vi "Check Stop.vi"(5 "VolatusAPI":refnum<class "VolatusAPI.lvclass">, 6 "State Loop Data in":T1, 7 "State Control":T9, 11 "State in":refnum<class "State.lvclass">) -> (1 "Stop":bool, 3 "State out":refnum<class "State.lvclass">, 4 "State Loop Data":T1)   [LabVIEW 2023, in "VolatusSeq.lvlib" / "State.lvclass"]
uses:
  State.lvclass
  State Control.ctl
  Sequence Time.ctl
  Variables/Variables.lvclass
  State Loop Data.ctl
  Iteration Actions/Iteration Actions.lvclass
  Command.ctl
  Volatus/MessageQ/MessageQ.lvclass
  Format String/Format String.lvclass
  VolatusSeqConfig/Command Type.ctl
  messages/CmdDigital/Data.ctl
  messages/CmdAnalog/Data.ctl
  Send Type.ctl
  lv-vecto/Vecto/Channel DBL/Channel DBL.lvclass
  Transition/Transition.lvclass
  VolatusSeqConfig/Debug Flags.ctl
  Volatus/VolatusAPI/VolatusAPI.lvclass
  State.lvclass/State.ctl
  Iteration Actions/Iteration Actions.lvclass/Iteration Actions.ctl
  VolatusSeq.lvlib
  VolatusSeqConfig/VolatusSeqConfig.lvlib
  messages/CmdDigital/CmdDigital.lvlib
  messages/CmdAnalog/CmdAnalog.lvlib
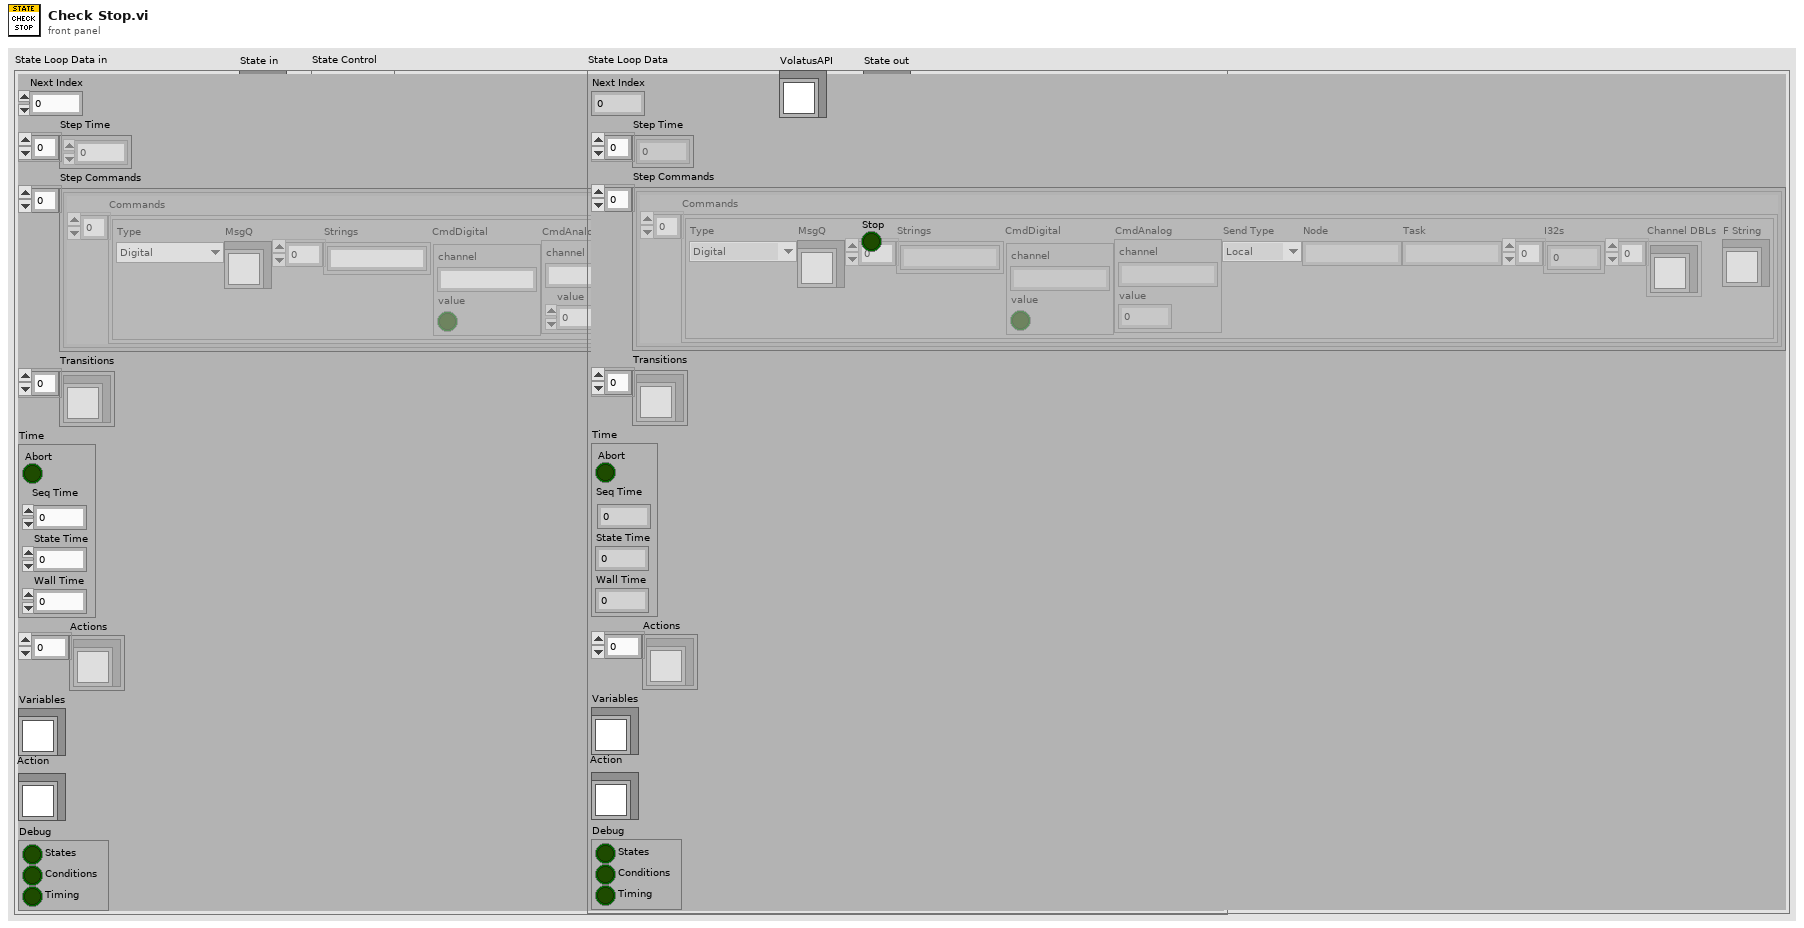
[diagram p1: front panel]
types:
  T1 = typedef "VolatusSeq.lvlib/State.lvclass/State Loop Data.ctl" = cluster{"Next Index":i32, "Step Time":dbl[], "Step Commands":cluster{"Commands":T2[]}[], "Transitions":refnum<class "Transition.lvclass">[], "Time":T7, "Actions":refnum<class "Iteration Actions.lvclass">[], "Variables":refnum<class "Variables.lvclass">, "Action":refnum<class "Iteration Actions.lvclass">, "Debug":T8}
  T2 = typedef "VolatusSeq.lvlib/Command.ctl" = cluster{"Type":T3, "MsgQ":refnum<class "MessageQ.lvclass">, "Strings":string[], "CmdDigital":T4, "CmdAnalog":T5, "Send Type":T6, "Node":string, "Task":string, "I32s":i32[], "Channel DBLs":refnum<class "Channel DBL.lvclass">[], "F String":refnum<class "Format String.lvclass">}
  T3 = typedef "VolatusSeqConfig.lvlib/Command Type.ctl" = enum16{"Digital", "Numeric", "Transition", "Stop", "StartLog", "StopLog", "Start", "Event", "Error", "HTTP", "ResetVar", "IncVar", "DecVar", "SaveVar", "LoadVar", "AddVar", "SubVar", "SetVar", "AddToVar"}
  T4 = typedef "CmdDigital.lvlib/Data.ctl" = cluster{"channel":string, "value":bool}
  T5 = typedef "CmdAnalog.lvlib/Data.ctl" = cluster{"channel":string, "value":dbl}
  T6 = typedef "VolatusSeq.lvlib/Send Type.ctl" = enum16{"Local", "Remote"}
  T7 = typedef "VolatusSeq.lvlib/Sequence Time.ctl" = cluster{"Abort":bool, "Seq Time":dbl, "State Time":dbl, "Wall Time":dbl}
  T8 = typedef "VolatusSeqConfig.lvlib/Debug Flags.ctl" = cluster{"States":bool, "Conditions":bool, "Timing":bool}
  T9 = typedef "VolatusSeq.lvlib/State Control.ctl" = cluster{"State":refnum<notifier>, "Time":refnum<notifier>, "Request State":refnum<notifier>, "Abort":refnum<notifier>, "Reset":refnum<notifier>, "Close":refnum<notifier>, "Vars SEQ":refnum<queue>}
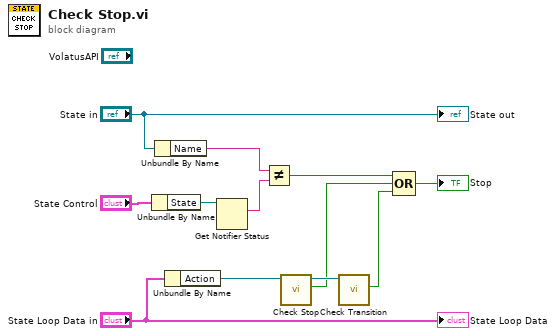
[diagram p0: block diagram]
diagram:
  n1 = Unbundle By Name("State Control") -> ("State"=w11:refnum<notifier>)
  n2 = Unbundle By Name("State in") -> ("Name"=w9:string)
  n3 = Unbundle By Name("State Loop Data in") -> ("Action"=w5:refnum<class "Iteration Actions.lvclass">)
  n4 = Get Notifier Status(notifier=w11) -> (current notification=w10:string)  [unwired: 1 in, 4 out]
  n5 = Not Equal?(x=w9, y=w10) -> (x != y?=w8:bool)
  n6 = call "Check Stop.vi"("Iteration Actions in"=w5) -> ("Stop Seq"=w1:bool, "Iteration Actions out"=w2:refnum<class "Iteration Actions.lvclass">)  [unwired: 8 in, 1 out]
  n7 = call "Check Transition.vi"("Iteration Actions in"=w2) -> ("Transition"=w3:bool)  [unwired: 7 in, 3 out]
  n8 = Compound Arithmetic op=OR(w8, w1, w3) -> (→"Stop":bool)
  "State out" <- "State in"
  "State Loop Data" <- "State Loop Data in"
